vi "BLED1112_app-connection.vi"(0 "COM Bluegiga in":refnum<visa-resource-name>="COM8", 1 "Device List":refnum<vi>, 5 "MAC Address":string="D9:2F:10:92:34:F2", 7 "Address Type":enum16{"Public", "Random"}(ring)=enum."Random", 9 "Conn Try no":i32=5, 11 "error in":errorcluster, 12 "discovery":refnum<vi>) -> (4 "COM out":refnum<visa-resource-name>="COM8", 6 "Connection Ok":bool=TRUE, 8 "Device Name":string="JUN_JUN", 10 "Handle table":string[][](array[string])=[["0001", "1800", "2800"], ["0002", "1800", "2803"], ["0003", "1800", "2A00"], ["0004", "1800", "2803"], ["0005", "1800", "2A01"], ["0006", "1800", "2803"], ["0007", "1800", "2A04"], ["0008", "1801", "2800"], ["0009", "0000F00D1212EFDE1523785FEF13D123", "2800"], ["000A", "0000F00D1212EFDE1523785FEF13D123", "2803"], ["000B", "0000F00D1212EFDE1523785FEF13D123", "000000011212EFDE1523785FEF13D123"], ["000C", "0000F00D1212EFDE1523785FEF13D123", "2902"], ["000D", "000000021212EFDE1523785FEF13D123", "2800"], ["000E", "000000021212EFDE1523785FEF13D123", "2803"], ["000F", "000000021212EFDE1523785FEF13D123", "000000021212EFDE1523785FEF13D123"], ["0010", "000000021212EFDE1523785FEF13D123", "2902"]], 14 "Connection Status":T1={"MAC Address"="D9:2F:10:92:34:F2", "cnx handle"=0, "cnx flags"=5, "Address Type"=1, "Connection Interval (ms)"=15, "Timeout(ms)"=1000, "Latency"=0, "bonding handle"=255} {"Address Type" items=["Public", "Random"]}, 15 "에러 출력":errorcluster={"status"=FALSE, "code"=1073676294, "source"="ble_read_message.vi->ble_read_specific_message.vi->ble_evt_attclient_procedue_completed.vi->ble_write_by_handle_uint8array.vi->ble_write_by_service_characteristic_uint8array.vi->BLED1112_app-connection.vi->[BLE Test] ble_read_write_characteristics.vi 안에 VISA 읽기"})   [LabVIEW 2015]
uses:
  Lib_Bled112 toolkit/type_def/connection_status_bundle.ctl
  Lib_Bled112 toolkit/type_def/address_type.ctl
  Lib_Bled112 toolkit/ble_functions/ble_write_by_service_characteristic_uint8array.vi
panel:
  out "Conn try":i32=4
  out "Get Device name?":bool=TRUE
  out "Get handle table?":bool=TRUE
  out "Connected?":bool=TRUE
  # "BLE Connection"
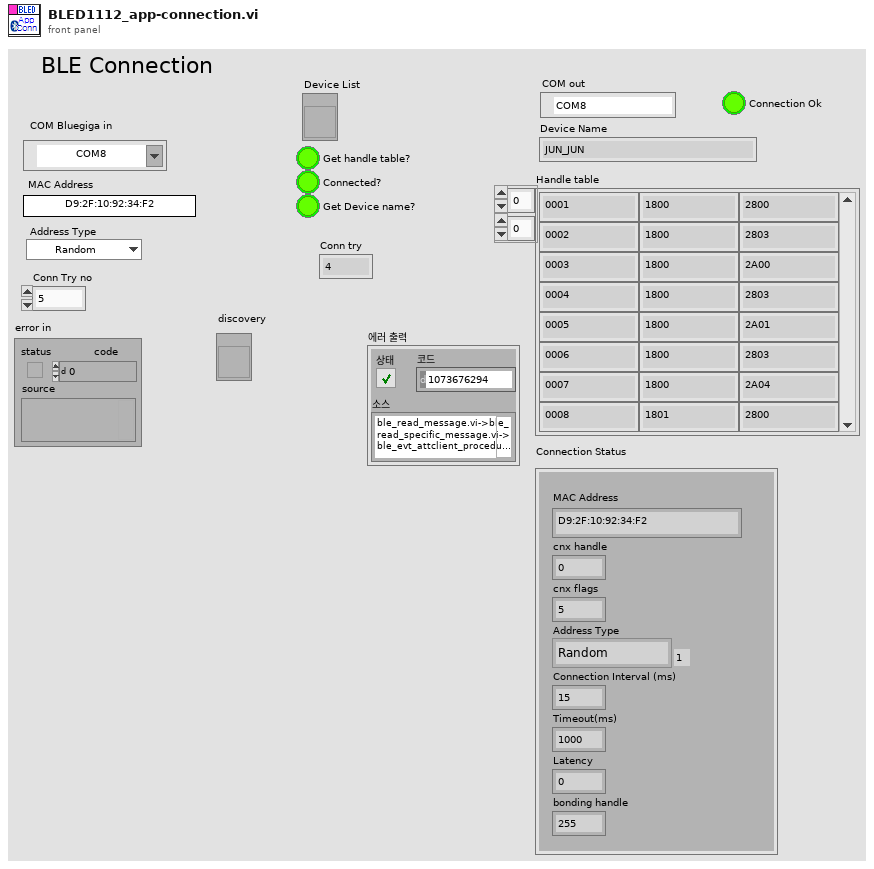
[diagram p1: front panel]
types:
  T1 = typedef "connection_status_bundle.ctl" = cluster{"MAC Address":string, "cnx handle":u8, "cnx flags":u8, "Address Type":T2, "Connection Interval (ms)":u16, "Timeout(ms)":u16, "Latency":u16, "bonding handle":u8}
  T2 = typedef "address_type.ctl" = u8
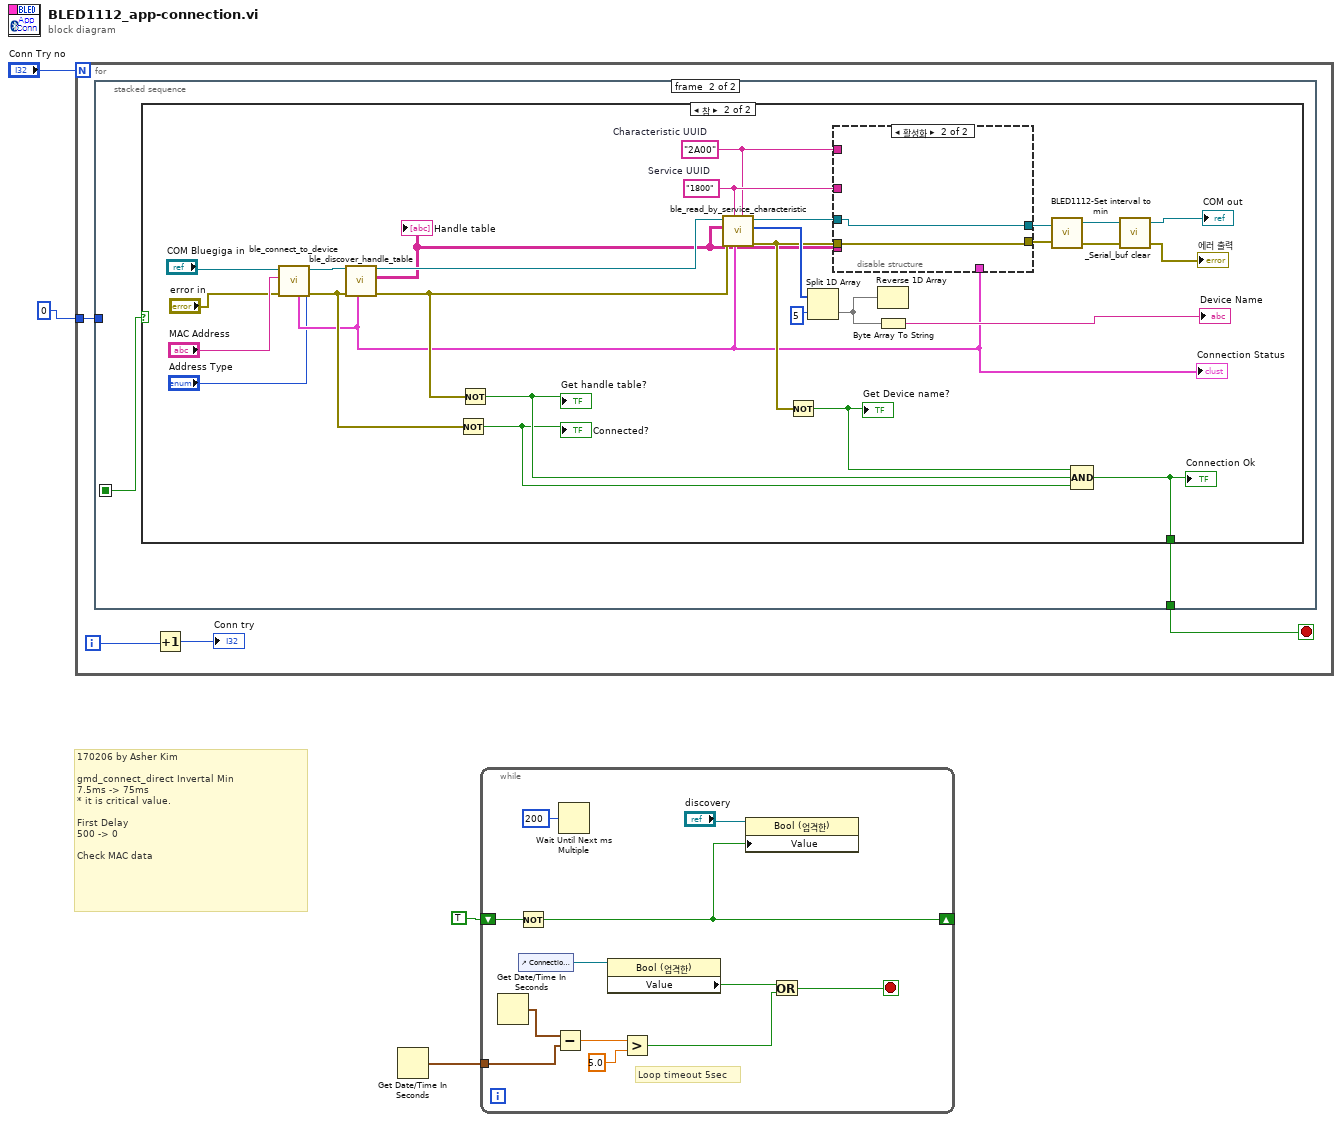
[diagram p0: block diagram]
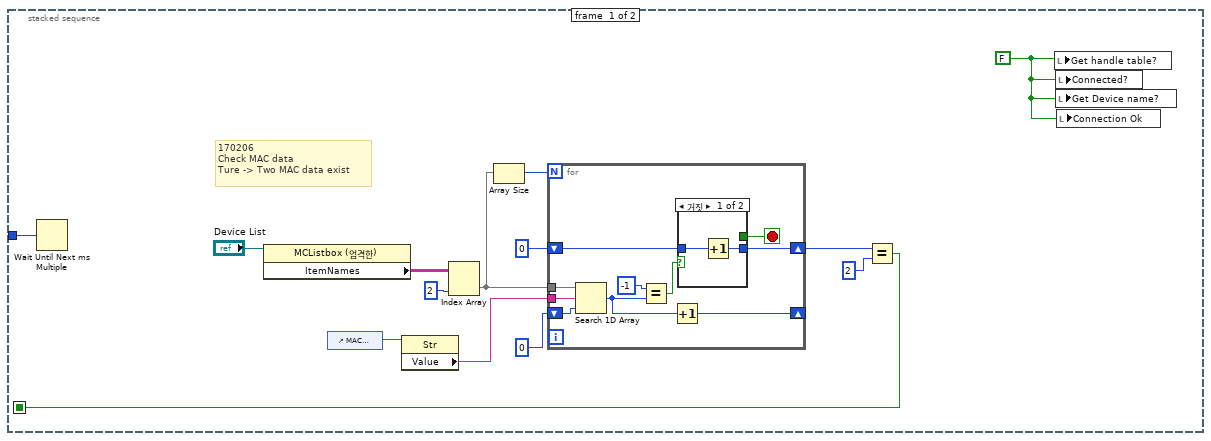
[diagram p2: hidden frame]
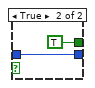
[diagram p3: hidden frame]
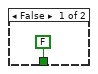
[diagram p4: hidden frame]
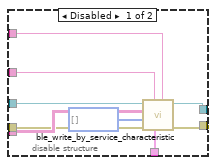
[diagram p5: hidden frame]
diagram:
  # "170206 by Asher Kim\n\ngmd_connect_direct Invertal Min\n7.5ms -> 75ms\n* it is critical value.\n\nFirst Delay\n500 -> 0\n\nCheck MAC data"
  n1 = for {
    N: "Conn Try no" -> [_]
    tunnel: u32 0 ("ms 배수") -> [w8]
    i -> [w5]
    stop <- w7 stop-if-true
    n2 = stacked-sequence {
      seq-local: [w9 _] -> [_ w37]
      tunnel: [_ w38] -> w7
      tunnel: w8 -> [w22 _]
      frame #0 {
        w21 = FALSE ("Get handle table?")
        # "170206\nCheck MAC data\nTure -> Two MAC data exist"
        n3 = Wait Until Next ms Multiple(millisecond multiple=w22) -> ()  [unwired: 1 out]
        n4 = property class="MCListbox (엄격한)"(reference="Device List") -> ("ItemNames"=w12:string[][])  [unwired: 1 in, 2 out]
        n5 = control-ref of="MAC Address"() -> (w19:refnum<vi>)
        n6 = property class="Str"(reference=w19) -> ("Value"=w13:string)  [unwired: 1 in, 2 out]
        n7 = Index Array(array=w12, index (col)=2 ("비활성화된 인덱스 (열)")) -> (element=w17:string[])  [unwired: 1 in]
        n8 = Array Size(array=w17) -> (size(s)=w16:i32)
        n9 = for {
          N: w16 -> [_]
          tunnel: w17 -> [w32]
          tunnel: w13 -> [w31]
          shift-right: [w27] -> _
          shift-left: 0 ("index of element") -> [w28]
          shift-right: [w29] -> w11
          shift-left: 0 ("index of element") -> [w30]
          stop <- w23 stop-if-true
          n10 = Search 1D Array(1D array=w32, element=w31, start index (0)=w28) -> (index of element=w26:i32)
          n11 = Equal?(x=-1, y=w26) -> (x = y?=w25:bool)
          n12 = Increment(x=w26) -> (x+1=w27:i32)
          n13 = case shown="거짓" w25 {
            tunnel: w30 -> [w34 w36]
            tunnel: [w33 w36] -> w29
            tunnel: [_ TRUE] -> w23
            frame False {
              n14 = Increment(x=w34) -> (x+1=w33:i32)
            }
            frame True {
            }
          }
        }
        n15 = Equal?(x=w11, y=2) -> (x = y?=w9:bool)
        n16 = local write "Get handle table?"(w21) -> ()
        n17 = local write "Connected?"(w21) -> ()
        n18 = local write "Get Device name?"(w21) -> ()
        n19 = local write "Connection Ok"(w21) -> ()
      }
      frame #1 {
        n20 = case shown="참" w37 {
          tunnel: [FALSE w40] -> w38
          frame False {
          }
          frame True {
            w62 = "2A00"  # Characteristic UUID
            w63 = "1800"  # Service UUID
            n21 = call "ble_connect_to_device.vi"("Address Type"="Address Type", "error in (no error)"="error in", "MAC Address"="MAC Address", "COM Bluegiga in"="COM Bluegiga in") -> ("error out"=w58:errorcluster, "COM Bluegiga out"=w59:refnum<visa-resource-name>, "Connection Status"=w51:T1)  [unwired: 5 in]
            "Connection Status" <- w51
            n22 = call "ble_discover_handle_table.vi"("Connection Status"=w51, "error in (no error)"=w58, "COM Bluegiga in"=w59) -> ("error out"=w57:errorcluster, "Handle table"=w42:string[][], "COM Bluegiga out"=w67:refnum<visa-resource-name>)  [unwired: 6 in]
            "Handle table" <- w42
            n23 = Not(x=w58) -> (.not. x?=w43:bool)
            "Connected?" <- w43
            n24 = Not(x=w57) -> (.not. x?=w44:bool)
            "Get handle table?" <- w44
            n25 = call "ble_read_by_service_characteristic.vi"("Characteristic UUID"=w62, "Connection Status"=w51, "Service UUID"=w63, "error in (no error)"=w57, "Handle table"=w42, "COM Bluegiga in"=w67) -> ("error out"=w56:errorcluster, "characteristic value"=w61:u8[], "COM Bluegiga out"=w64:refnum<visa-resource-name>)  [unwired: 3 in]
            n26 = Not(x=w56) -> (.not. x?=w45:bool)
            "Get Device name?" <- w45
            n27 = Split 1D Array(array=w61, index=5) -> (second subarray=w60:u8[])  [unwired: 1 out]
            n28 = disable-structure shown="활성화" {
              disable-tunnel: w64 -> [w76 w78]
              disable-tunnel: w63 -> [w75 _]
              disable-tunnel: w62 -> [w74 _]
              disable-tunnel: w42 -> [w73 _]
              disable-tunnel: w56 -> [w72 w77]
              disable-tunnel: [w71 w78] -> w55
              disable-tunnel: [w70 w77] -> w54
              disable-tunnel: w51 -> [w69 _]
              frame Disabled {
                n29 = call-poly "ble_write_by_service_characteristic.vi"("Characteristic UUID"=w74, "Connection Status"=w69, "Service UUID"=w75, "error in (no error)"=w72, "data"=u8[] [], "Handle table"=w73, "COM Bluegiga in"=w76) -> ("error out"=w70:errorcluster, "COM Bluegiga out"=w71:refnum<visa-resource-name>)  [unwired: 3 in]
              }
              frame Enabled {
              }
            }
            n30 = Reverse 1D Array(array=w60) -> ()  [unwired: 1 out]
            n31 = Byte Array To String(unsigned byte array=w60) -> (string=→"Device Name":string)
            n32 = call "BLED1112-Set interval to min.vi"("에러 입력(에러 없음)"=w54, "VISA 리소스 이름"=w55) -> ("에러 출력"=w52:errorcluster, "VISA 리소스 이름 출력"=w53:refnum<visa-resource-name>)
            n33 = Compound Arithmetic op=AND ("복합 연산")(w45, w44, w43) -> (w40:bool)
            "Connection Ok" <- w40
            n34 = call "_Serial_buf clear.vi"("에러 출력 2"=w52, "Serial Port"=w53) -> ("에러 출력"=→"에러 출력":errorcluster, "Serial Port 2"=→"COM out":refnum<visa-resource-name>)  [unwired: 2 in]
          }
        }
      }
    }
    n35 = Increment(x=w5) -> (x+1=→"Conn try":i32)
  }
  n36 = Get Date/Time In Seconds() -> (seconds since 1Jan1904=w1:timestamp)
  n37 = while {
    shift-right: [w87] -> _
    shift-left: TRUE -> [w88]
    tunnel: w1 -> [w83]
    stop <- w84 stop-if-true
    # "Loop timeout 5sec"
    n38 = Get Date/Time In Seconds() -> (seconds since 1Jan1904=w79:timestamp)
    n39 = Not(x=w88) -> (.not. x?=w87:bool)
    n40 = control-ref of="Connection Ok"() -> (w86:refnum<vi>)
    n41 = Subtract(x=w79, y=w83) -> (x-y=w82:dbl)
    n42 = Wait Until Next ms Multiple(millisecond multiple=u32 200 ("ms 배수")) -> ()  [unwired: 1 out]
    n43 = property class="Bool (엄격한)"(reference=w86) -> ("Value"=w85:bool)  [unwired: 1 in, 2 out]
    n44 = Greater?(x=w82, y=5.0) -> (0:w80:bool)
    n45 = property class="Bool (엄격한)"(reference="discovery", "Value"=w87) -> ()  [unwired: 1 in, 2 out]
    n46 = Or(x=w85, y=w80) -> (x .or. y?=w84:bool)
  }
